vi "CC_PI_MAIN_TESTING.vi"() -> ()   [LabVIEW 2019]
uses:
  <vilib>/FPGAPlugInAG/sbRIO-9627/niLvFpga_Open_sbRIO-9627.vi
  <vilib>/rvi/interface/common/dynamic/niFpgaDynamicAddResources.vi
  <vilib>/Utility/error.llb/Error Cluster From Error Code.vi
  <vilib>/rvi/errors/niLvFpgaAdjustHostInterfaceError.vi
  <vilib>/FPGAPlugInAG/Dynamic/niLvFpga_Close_Dynamic.vi
  <vilib>/rvi/interface/nirviOpenFPGA/nirviOpenFPGA.xnode
  FPGA Bitfiles/ccmultiplier_FPGATarget_CCPItesting_ybhjPyRilUw.lvbitx
  CC_PI_testing.vi
  <vilib>/rvi/interface/nirviReadWriteControl/nirviReadWriteControl.xnode
  <vilib>/rvi/interface/nirviCloseFPGA/nirviCloseFPGA.xnode
  NiFpgaLv.dll
  <vilib>/rvi/interface/Simulation/niFpgaSimulationCallBeginRW.vi
panel:
  out "error %":sgl(knob) scale=-100.0..100.0
  out "Loop rate":u16
  in  "Kp":sgl
  in  "Ki":sgl
  in  "zero Value motor":sgl
  in  "weighting term motor":sgl
  in  "Fre":sgl
  in  "amplitude":sgl
  in  "stop":bool
  out "Current control":dynamicdata(graph)
  out "motor direction":bool
  out "control_ip":sgl(graph)
  out "raw current":sgl(graph)
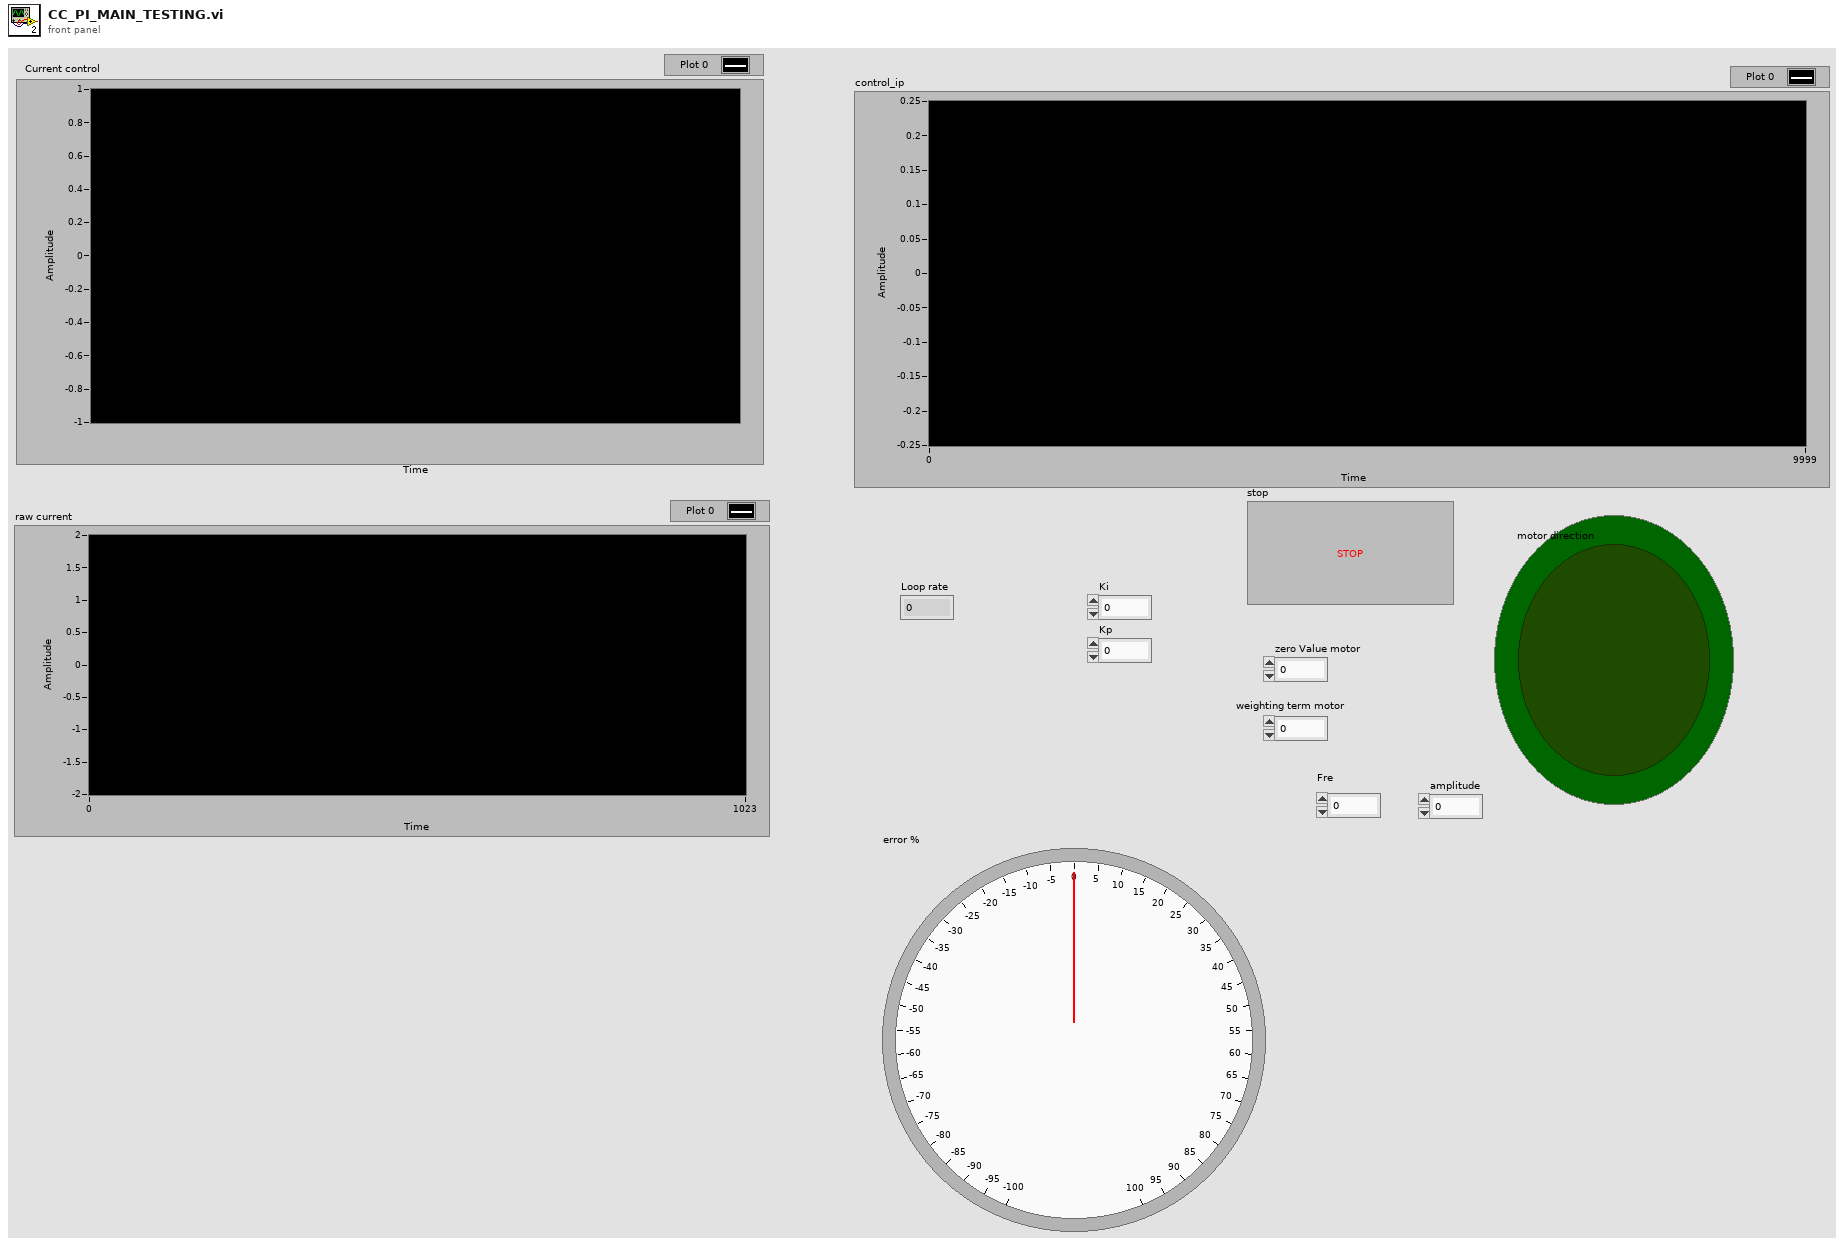
[diagram p1: front panel]
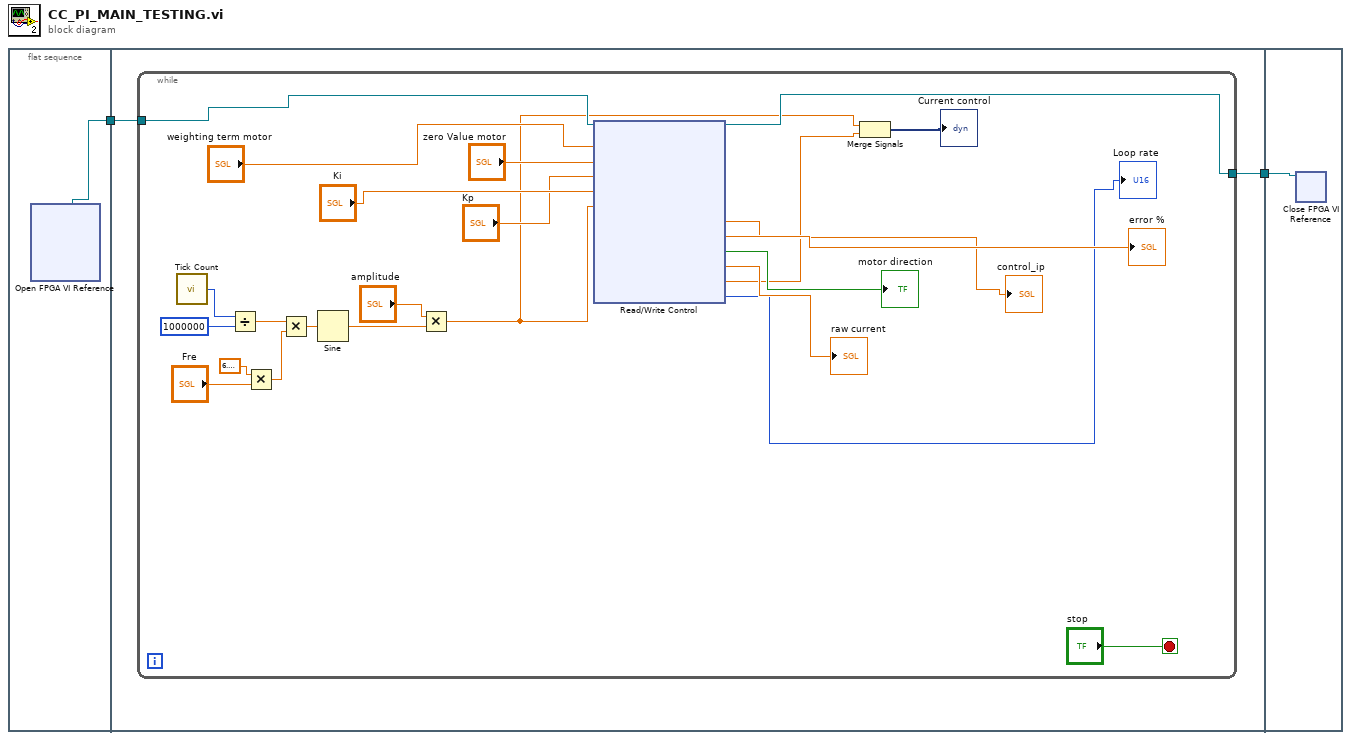
[diagram p0: block diagram]
diagram:
  n1 = flat-sequence {
    tunnel: [w3] -> w2
    tunnel: w2 -> [w5]
    tunnel: [w4] -> w1
    tunnel: w1 -> [w30]
    frame #0 {
      n2 = xnode "Open FPGA VI Reference"() -> ("FPGA VI Reference Out"=w3:refnum<k20>)  [unwired: 2 in, 1 out]
    }
    frame #1 {
      n3 = while {
        tunnel: w5 -> [w18]
        tunnel: [w17] -> w4
        stop <- "stop" stop-if-true
        n4 = call "Tick Count"() -> ("Tick Count(uSec)"=w29:u32)
        n5 = Divide(x=w29, y=u32 1000000) -> (x/y=w22:dbl)
        n6 = Multiply(x=sgl 6.2831855, y="Fre") -> (x*y=w27:sgl)
        n7 = Multiply(x=w22, y=w27) -> (x*y=w26:dbl)
        n8 = Sine(x=w26) -> (sin(x)=w23:dbl)
        n9 = Multiply(x="amplitude", y=w23) -> (x*y=w7:dbl)
        n10 = xnode "Read/Write Control"("FPGA VI Reference In"=w18, "weighting term(M2)"="weighting term motor", "zero Value M2"="zero Value motor", "Kp"="Kp", "Ki"="Ki", "reference"=w7) -> ("FPGA VI Reference Out"=w17:refnum<k20>, "control_ip"=→"control_ip":sgl, "error %"=→"error %":sgl, "motor direction"=→"motor direction":bool, "raw current"=→"raw current":sgl, "Filtered Current(M2)"=w6:sgl, "Loop rate"=→"Loop rate":u16)  [unwired: 1 in, 1 out]
        n11 = Merge Signals(w7, w6) -> (→"Current control":dynamicdata)
      }
    }
    frame #2 {
      n12 = xnode "Close FPGA VI Reference"("FPGA VI Reference In"=w30) -> ()  [unwired: 1 in, 1 out]
    }
  }
